vi "Write local path.vi"(8 "error in":errorcluster, 10 "local path":path, 11 "Shared Library Module editor node in":refnum<class "Shared Library Module editor node.lvclass">) -> (0 "error out":errorcluster, 3 "Shared Library Module editor node out":refnum<class "Shared Library Module editor node.lvclass">)   [LabVIEW 2013, in "Shared Library Module editor node.lvclass"]
uses:
  Shared Library Module editor node.lvclass
  <vilib>/NI/DCAF/Tag Editor Core/Configuration Editor/Classes/Module editor node/module editor node.lvclass
  <vilib>/NI/Configuration Framework/serializable configuration/NISE_CEF_serializable configuration.lvclass
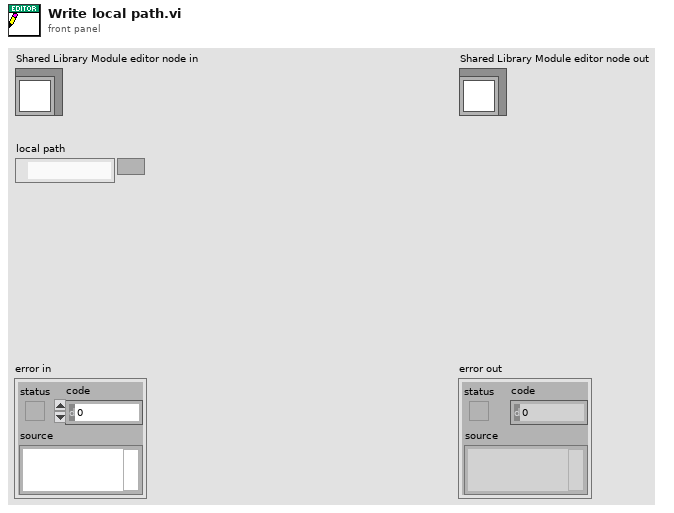
[diagram p1: front panel]
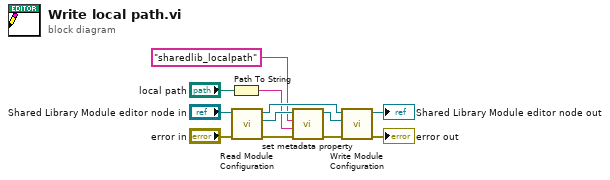
[diagram p0: block diagram]
diagram:
  n1 = Path To String(path="local path") -> (string=w1:string)
  n2 = call <vilib>:"Read Module Configuration.vi"("error in"="error in", "Module Editor Node in"="Shared Library Module editor node in") -> ("error out"=w6:errorcluster, "module configuration"=w7:refnum<class "TBM module configuration.lvclass">, "Module Editor Node out"=w11:refnum<class "Shared Library Module editor node.lvclass">)  [unwired: 7 in]
  n3 = call <vilib>:"set metadata property.vi"("error in"=w6, "value"=w1, "key"="sharedlib_localpath", "configuration in"=w7) -> ("error out"=w4:errorcluster, "configuration out"=w5:refnum<class "TBM module configuration.lvclass">)  [unwired: 6 in]
  n4 = call <vilib>:"Write Module Configuration.vi"("error in"=w4, "module configuration"=w5, "Module Editor Node in"=w11) -> ("error out"=→"error out":errorcluster, "Module Editor Node out"=→"Shared Library Module editor node out":refnum<class "Shared Library Module editor node.lvclass">)  [unwired: 7 in]
